vi "Motor Control Enhanced.vi"(0 "PID On":bool) -> (5 "Total (V)":dbl[](array[slide]) scale=-8.0..8.0, 6 "Force (N)":T2(graph)={"M1 ref force"=20.0, "M2 ref force"=20.0, "M1 mes force"=0.47897514031400124, "M2 mes force"=1.2484368104304875})   [LabVIEW 2021]
uses:
  <vilib>/Platform/TimedLoop/XDataNode/timing_clust.ctl
  <vilib>/Platform/TimedLoop/XDataNode/nitl_modes.ctl
  <vilib>/Platform/TimedLoop/XDataNode/wakeup.ctl
  <vilib>/DAQmx/write.llb/DAQmx Write (Digital 1D Bool 1Chan 1Samp).vi
  <vilib>/DAQmx/write.llb/DAQmx Write (Analog 1D DBL NChan 1Samp).vi
  <vilib>/DAQmx/create/channels.llb/DAQmx Create Channel (DO-Digital Output).vi
  <vilib>/DAQmx/create/channels.llb/DAQmx Create Channel (AO-Voltage-Basic).vi
  <vilib>/DAQmx/create/channels.llb/DAQmx Create Channel (AI-Voltage-Basic).vi
  <vilib>/DAQmx/miscellaneous.llb/DAQmx Fill In Error Info.vi
  <vilib>/Platform/TimedLoop/XDataNode/XDataNode.xnode
  <vilib>/Platform/TimedLoop/XDataNode/XDNodeRunTimeDep.lvlib
panel:
  in  "s":bool
  in  "Numeric":dbl
  in  "Tab Control":enum32{"PID Gain", "PIN On"}(tab)=enum."PIN On"
  in  "Gains":T1(array[cluster])=[{"proportional gain (Kc)"=0.17, "integral time (Ti, min)"=0.0, "derivative time (Td, min)"=0.0}, {"proportional gain (Kc)"=0.17, "integral time (Ti, min)"=0.0, "derivative time (Td, min)"=0.0}] {"derivative time (Td, min)" format="%.3f"; "integral time (Ti, min)" format="%.3f"; "proportional gain (Kc)" format="%.3f"}
  out "PID (V)":dbl[](array[slide])=[3.31857422614662, 1.0] scale=-8.0..8.0
  out "Trigger":bool
  in  "Loadcell":bool
  in  "Encoder":bool
  out "Speed (RPM)":dbl[](array[knob]) scale=-200.0..200.0
  out "time (s)":dbl=642.808
  in  "Set Point":dbl(slide)=19.814241486068113 scale=0.0..40.0
  in  "Motor Enable":bool[](array[boolean])=[FALSE, FALSE]
  in  "stop":bool
  # "Gait"
  # "Balance"
  # "INITIALIZE"
  # "TUNE"
  # "MONITOR"
  # "DEVEL"
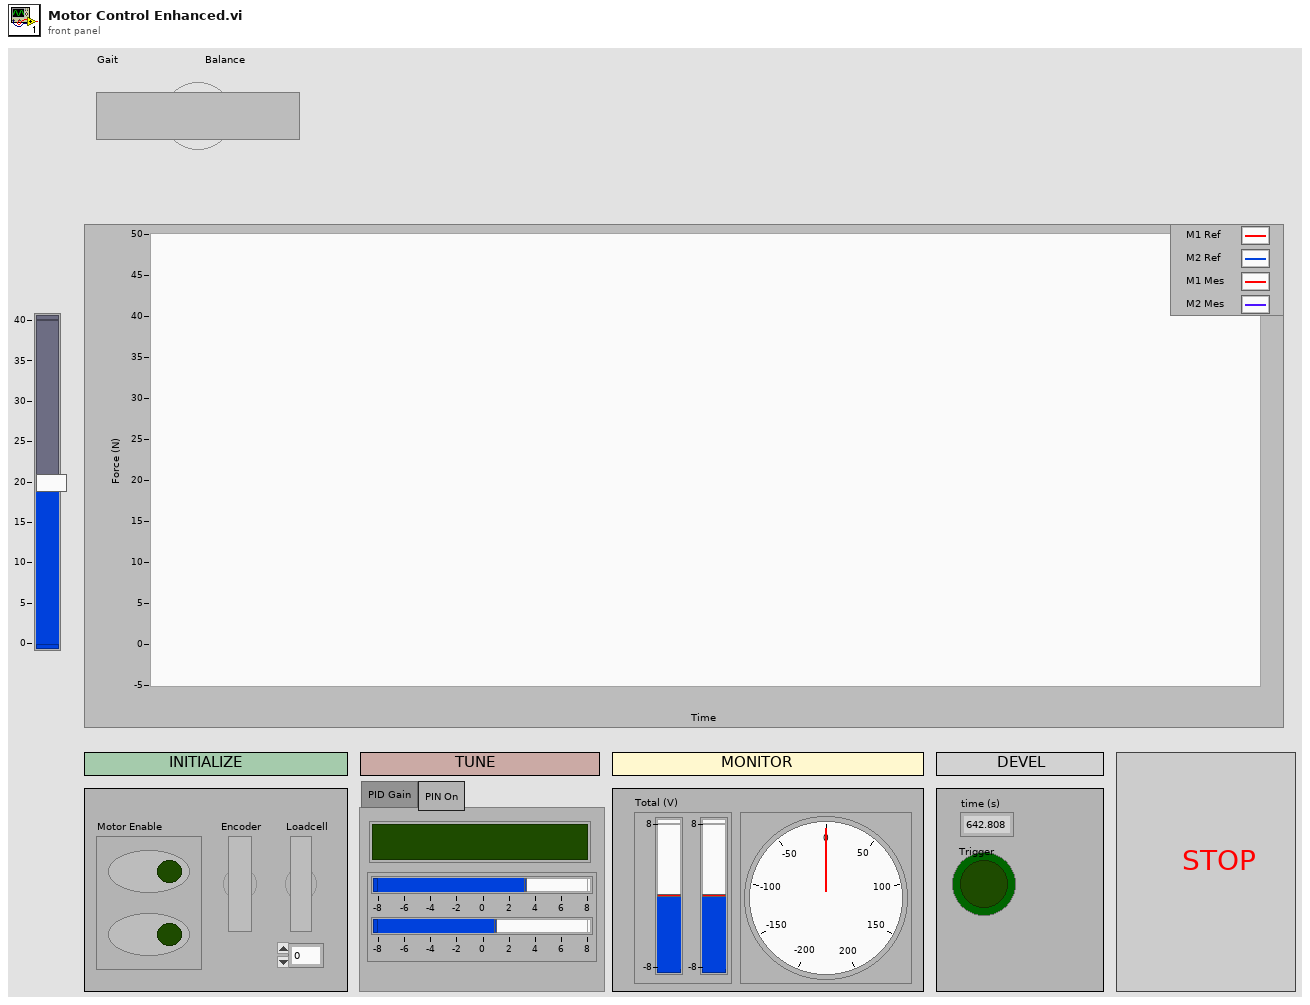
[diagram p1: front panel]
types:
  T1 = cluster{"proportional gain (Kc)":dbl, "integral time (Ti, min)":dbl, "derivative time (Td, min)":dbl}[]
  T2 = cluster{"M1 ref force":dbl, "M2 ref force":dbl, "M1 mes force":dbl, "M2 mes force":dbl}
  T3 = typedef "XDNodeRunTimeDep.lvlib/timing_clust.ctl" = cluster{"Expected End [f-1]":u64, "Actual End [f-1]":u64, "Finished Late? [f-1]":bool, "Expected End [i-1]":u64, "Actual End [i-1]":u64, "Finished Late? [i-1]":bool, "Expected Start [i]":u64, "Actual Start [i]":u64, "Expected Start [f]":u64, "Actual Start [f]":u64, "Source Name":string, "Structure Name":string, "Period":i64, "Deadline":i64, "Offset":i64, "Start":i64, "Priority":i32, "Timeout":i32, "Mode":T4, "Wakeup Reason":T5, "Error":errorcluster, "Source Type":string, "Secondary Source Type":string, "Global End Time":u64, "Global Start Time":u64, "Frame Duration":u64, "Iteration Duration":u64, "Assigned CPU":i32, "I/O Scan Engine Mode":u32}
  T4 = typedef "XDNodeRunTimeDep.lvlib/nitl_modes.ctl" = enum32{"No Change", "Process missed periods, maintain original phase", "Discard missed periods, maintain original phase", "Process missed periods, ignore original phase", "Discard missed periods, ignore original phase"}
  T5 = typedef "XDNodeRunTimeDep.lvlib/wakeup.ctl" = enum32{"Normal", "Aborted", "Asynchronous wakeup", "Timing source error", "Timed loop error", "Timeout"}
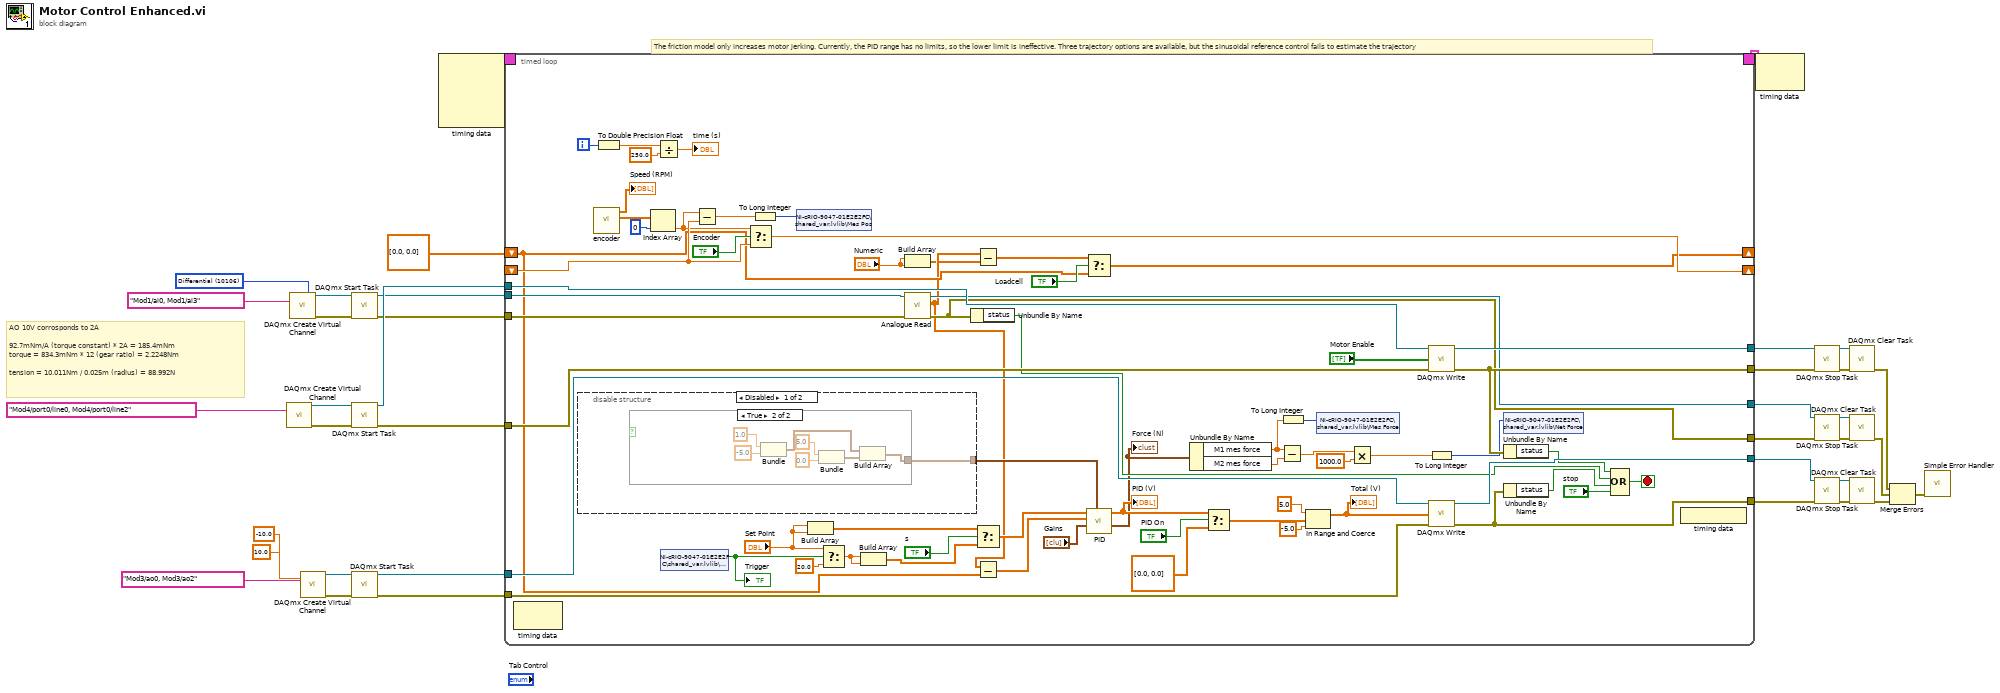
[diagram p0: block diagram]
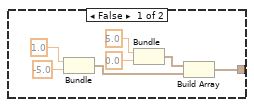
[diagram p2: hidden frame]
diagram:
  w2 = 10106 items=["Default"=-1, "RSE"=10083, "NRSE"=10078, "Differential"=10106, "Pseudodifferential"=12529] ("input terminal configuration")
  # "The friction model only increases motor jerking. Currently, the PID range has no limits, so the lower limit is ineffective. Three trajectory options are available, but the sinusoidal reference control fails to estimate the trajectory"
  # "AO 10V corrosponds to 2A\n\n92.7mNm/A (torque constant) * 2A = 185.4mNm\ntorque = 834.3mNm * 12 (gear ratio) = 2.2248Nm\n\ntension = 10.011Nm / 0.025m (radius) = 88.992N"
  n1 = call-poly <vilib>:"DAQmx Create Virtual Channel.vi"("lines"=tag "Mod4/port0/line0, Mod4/port0/line2") -> ("task out"=w29:refnum<k21>, "error out"=w28:errorcluster)  [unwired: 13 in]
  n2 = call-poly <vilib>:"DAQmx Create Virtual Channel.vi"("input terminal configuration"=w2, "physical channels"=tag "Mod1/ai0, Mod1/ai3") -> ("task out"=w19:refnum<k21>, "error out"=w20:errorcluster)  [unwired: 12 in]
  n3 = call-poly <vilib>:"DAQmx Create Virtual Channel.vi"("maximum value"=10.0 ("AO max"), "minimum value"=-10.0 ("AO min"), "physical channels"=tag "Mod3/ao0, Mod3/ao2" ("Physical Channel(s)")) -> ("task out"=w13:refnum<k21>, "error out"=w12:errorcluster)  [unwired: 11 in]
  n4 = call <vilib>:"DAQmx Start Task.vi"("task/channels in"=w19, "error in"=w20) -> ("task out"=w17:refnum<k21>, "error out"=w16:errorcluster)  [unwired: 12 in]
  n5 = call <vilib>:"DAQmx Start Task.vi"("task/channels in"=w29, "error in"=w28) -> ("task out"=w26:refnum<k21>, "error out"=w25:errorcluster)  [unwired: 12 in]
  n6 = call <vilib>:"DAQmx Start Task.vi"("task/channels in"=w13, "error in"=w12) -> ("task out"=w31:refnum<k21>, "error out"=w30:errorcluster)  [unwired: 12 in]
  n7 = node-c288() -> (w33:T3)  [unwired: 4 in]
  n8 = timed-loop {
    tunnel: [w101] -> w37
    tunnel: [w100] -> w36
    tunnel: [w65] -> w35
    tunnel: [w87] -> w34
    tunnel: w17 -> [w98]
    timing: w33 -> [_]
    timing-out: [_] -> w32
    tunnel: w16 -> [w97]
    tunnel: w31 -> [w64]
    tunnel: w30 -> [w99]
    tunnel: w26 -> [w96]
    tunnel: w25 -> [w95]
    tunnel: [w94] -> w22
    tunnel: [w88] -> w21
    shift-right: [w69] -> _
    shift-left: _ -> [w67]
    shift-right: [w53] -> _
    shift-left: dbl[] [0.0, 0.0] ("measured force") -> [w54]
    i -> [w76]
    stop <- w83 stop-if-true
    n9 = node-c288() -> ()  [unwired: 1 in, 1 out]
    n10 = disable-structure shown="Disabled" {
      disable-tunnel: [w102 _] -> w56
      frame Disabled {
        n11 = case shown="True" {
          selector: _ -> [_ _]
          tunnel: [w103 w110] -> w102
          frame False {
            n12 = Bundle(1.0, -5.0) -> (w108:cluster{dbl, dbl})  [unwired: 1 in]
            n13 = Bundle(5.0, 0.0) -> (w109:cluster{dbl, dbl})  [unwired: 1 in]
            n14 = Build Array(w109, w108) -> (w103:cluster{dbl, dbl}[])
          }
          frame True {
            n15 = Bundle(1.0, -5.0) -> (w111:cluster{dbl, dbl})  [unwired: 1 in]
            n16 = Bundle(5.0, 0.0) -> (w112:cluster{dbl, dbl})  [unwired: 1 in]
            n17 = Build Array(w111, w112) -> (w110:cluster{dbl, dbl}[])
          }
        }
      }
      frame Enabled {
      }
    }
    n18 = call "encoder.vi"() -> ("Mes Pos (mm)"=w71:dbl[], "RPM"=→"Speed (RPM)":dbl[])  [unwired: 10 in]
    n19 = To Double Precision Float(number=w76) -> (double precision float=w75:dbl)
    n20 = Index Array(array=w71, index=0) -> (element=w66:dbl)
    n21 = Divide(x=w75, y=250.0) -> (x/y=→"time (s)":dbl)
    n22 = shared-variable "NI-cRIO-9047-01E2E2FC\\shared_var.lvlib\\Trigger"() -> (w43:bool)  [unwired: 1 in, 1 out]
    "Trigger" <- w43
    n23 = Subtract(x=w66, y=w67) -> (x-y=w63:dbl)
    n24 = Select(t=w66, s="Encoder", f=w67) -> (s? t:f=w69:dbl)
    n25 = To Long Integer(number=w63) -> (32bit integer=w49:i32)
    n26 = shared-variable "NI-cRIO-9047-01E2E2FC\\shared_var.lvlib\\Mes Pos"(w49) -> ()  [unwired: 1 in, 1 out]
    n27 = Build Array("Set Point", "Set Point") -> (w38:dbl[])
    n28 = Select(t="Set Point", s=w43, f=20.0) -> (s? t:f=w41:dbl)
    n29 = Build Array(w41, w41) -> (w77:dbl[])
    n30 = Build Array("Numeric", "Numeric") -> (w44:dbl[])
    n31 = call "Analogue Read.vi"("error in"=w97, "task/channels in"=w98) -> ("error out"=w87:errorcluster, "measured force"=w51:dbl[], "task out"=w65:refnum<k21>)  [unwired: 6 in, 1 out]
    n32 = Unbundle By Name(w87) -> ("status"=w85:bool)
    n33 = Subtract(x=w51, y=w44) -> (x-y=w50:dbl[])
    n34 = Select(t=w38, s="s", f=w77) -> (s? t:f=w60:dbl[])
    n35 = Subtract(x=w51, y=w54) -> (x-y=w52:dbl[])
    n36 = Select(t=w50, s="Loadcell", f=w54) -> (s? t:f=w53:dbl[])
    n37 = call "PID.vi"("output range"=w56, "PID gains"="Gains", "mes force"=w52, "ref force"=w60) -> ("output cluster"=w46:T2, "PID output"=w81:dbl[])  [unwired: 6 in]
    "Force (N)" <- w46
    "PID (V)" <- w81
    n38 = Unbundle By Name(w46) -> ("M1 mes force"=w57:dbl, "M2 mes force"=w58:dbl)
    n39 = Select(t=w81, s="PID On", f=dbl[] [0.0, 0.0]) -> (s? t:f=w79:dbl[])
    n40 = Subtract(x=w57, y=w58) -> (x-y=w62:dbl)
    n41 = To Long Integer(number=w57) -> (32bit integer=w59:i32)
    n42 = In Range and Coerce(upper limit=5.0, x=w79, lower limit=-5.0) -> (coerced(x)=w89:dbl[])  [unwired: 1 out]
    "Total (V)" <- w89
    n43 = shared-variable "NI-cRIO-9047-01E2E2FC\\shared_var.lvlib\\Mes Force"(w59) -> ()  [unwired: 1 in, 1 out]
    n44 = Multiply(x=w62, y=1000.0) -> (x*y=w47:dbl)
    n45 = call-poly <vilib>:"DAQmx Write.vi"("task/channels in"=w96, "data"="Motor Enable", "error in"=w95) -> ("task out"=w94:refnum<k21>, "error out"=w88:errorcluster)  [unwired: 10 in, 1 out]
    n46 = To Long Integer(number=w47) -> (32bit integer=w48:i32)
    n47 = call-poly <vilib>:"DAQmx Write.vi"("task/channels in"=w64, "data"=w89, "error in"=w99) -> ("task out"=w101:refnum<k21>, "error out"=w100:errorcluster)  [unwired: 10 in, 1 out]
    n48 = shared-variable "NI-cRIO-9047-01E2E2FC\\shared_var.lvlib\\Net Force"(w48) -> ()  [unwired: 1 in, 1 out]
    n49 = Unbundle By Name(w88) -> ("status"=w84:bool)
    n50 = Unbundle By Name(w100) -> ("status"=w86:bool)
    n51 = Compound Arithmetic op=OR(w84, w85, w86, "stop") -> (w83:bool)
    n52 = node-c288() -> ()  [unwired: 1 out]
  }
  n53 = node-c288(w32) -> ()  [unwired: 1 out]
  n54 = call <vilib>:"DAQmx Stop Task.vi"("task/channels in"=w22, "error in"=w21) -> ("task out"=w24:refnum<k21>, "error out"=w23:errorcluster)  [unwired: 12 in]
  n55 = call <vilib>:"DAQmx Stop Task.vi"("task/channels in"=w35, "error in"=w34) -> ("task out"=w8:refnum<k21>, "error out"=w7:errorcluster)  [unwired: 12 in]
  n56 = call <vilib>:"DAQmx Stop Task.vi"("task/channels in"=w37, "error in"=w36) -> ("task out"=w10:refnum<k21>, "error out"=w9:errorcluster)  [unwired: 12 in]
  n57 = call <vilib>:"DAQmx Clear Task.vi"("task in"=w24, "error in"=w23) -> ("error out"=w3:errorcluster)  [unwired: 13 in]
  n58 = call <vilib>:"DAQmx Clear Task.vi"("task in"=w8, "error in"=w7) -> ("error out"=w4:errorcluster)  [unwired: 13 in]
  n59 = call <vilib>:"DAQmx Clear Task.vi"("task in"=w10, "error in"=w9) -> ("error out"=w5:errorcluster)  [unwired: 13 in]
  n60 = Merge Errors(w3, w4, w5) -> (w6:errorcluster)
  n61 = call <vilib>:"Simple Error Handler.vi"("error in (no error)"=w6) -> ()  [unwired: 4 in, 5 out]
